vi "Intake Button Read.vi"() -> ()   [LabVIEW 2015]
panel:
  out "Button Cluster":cluster{}
  out "D-Pad":T1
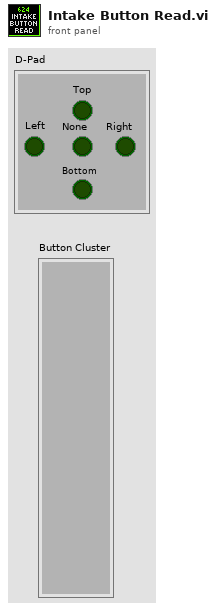
[diagram p1: front panel]
types:
  T1 = cluster{"None":bool, "Left":bool, "Bottom":bool, "Right":bool, "Top":bool}
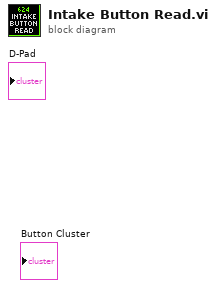
[diagram p0: block diagram]
diagram:
